vi "array2text.vi"(11 "Array":dbl[](array[numeric])) -> (3 "String":string)   [LabVIEW 2014]
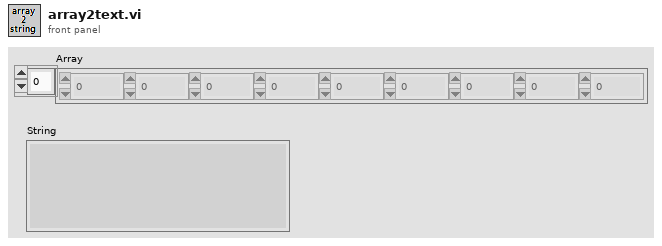
[diagram p1: front panel]
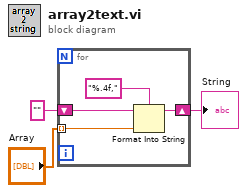
[diagram p0: block diagram]
diagram:
  n1 = for {
    tunnel: "Array" -> [w4] mode=indexing
    shift-right: [w6] -> w2
    shift-left: "" -> [w5]
    n2 = Format Into String(format string="%.4f,", initial string=w5, w4) -> (resulting string=w6:string)  [unwired: 1 in, 1 out]
  }
  "String" <- w2
